vi "Get CPU.vi"(8 "error in (no error)":errorcluster, 11 "Hardware Info in":refnum<class "Hardware Info.lvclass">) -> (0 "error out":errorcluster, 2 "CPU Info":refnum<class "CPU Info.lvclass">, 3 "Hardware Info out":refnum<class "Hardware Info.lvclass">)   [LabVIEW 2017, in "DSF Core.lvlib" / "Hardware Info.lvclass"]
uses:
  Hardware Info/Hardware Info.lvclass
  CPU Info/CPU Info.lvclass
  Hardware Info/Hardware Info.lvclass/Hardware Info.ctl
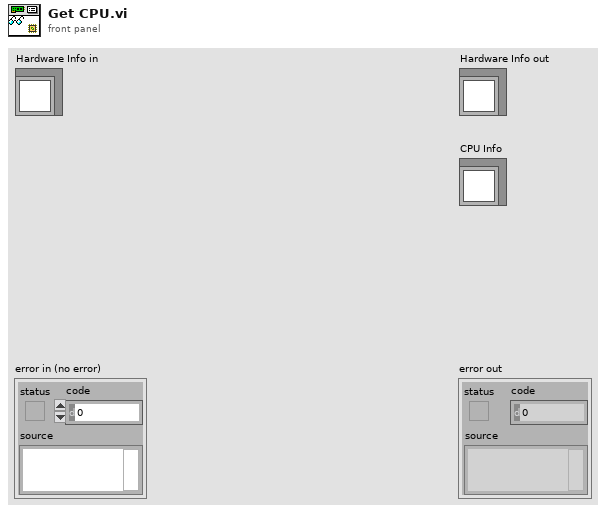
[diagram p1: front panel]
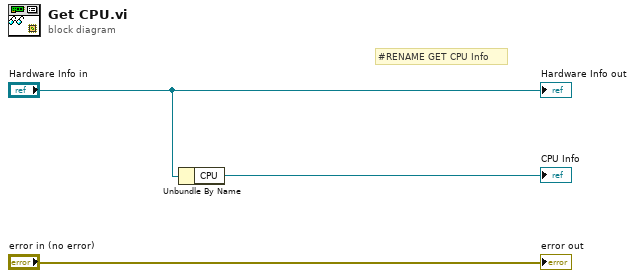
[diagram p0: block diagram]
diagram:
  # "#RENAME GET CPU Info"
  n1 = Unbundle By Name("Hardware Info in") -> ("CPU"=→"CPU Info":refnum<class "CPU Info.lvclass">)
  "error out" <- "error in (no error)"
  "Hardware Info out" <- "Hardware Info in"
